vi "XY Graph to Intensity Graph.vi"(8 "error in (no error)":errorcluster, 9 "Y Label":string, 10 "Y Scale":dbl[](array[numeric]), 11 "graph_utilities in":refnum<class "graph_utilities.lvclass">) -> (0 "error out":errorcluster, 3 "graph_utilities out":refnum<class "graph_utilities.lvclass">)   [LabVIEW 2019, in "graph_utilities.lvclass"]
uses:
  graph_utilities.lvclass
  XY Utilities/xy_utilities.lvlib
  XY Utilities/subVIs/Interpolate (multiple).vi
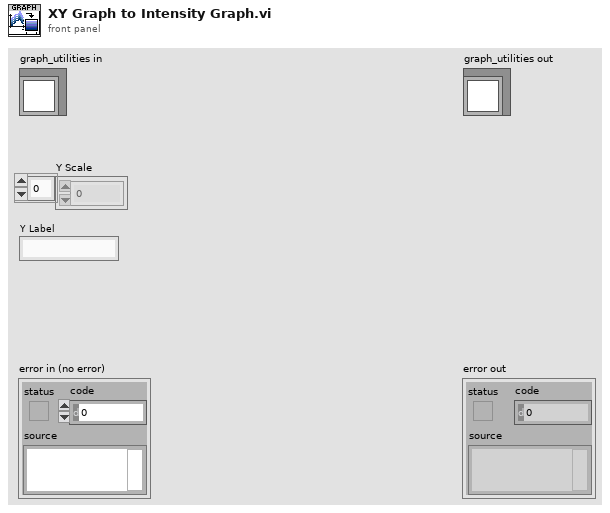
[diagram p1: front panel]
types:
  T1 = cluster{"X Low":dbl, "X High":dbl, "X Step":dbl, "Fake Point":dbl}
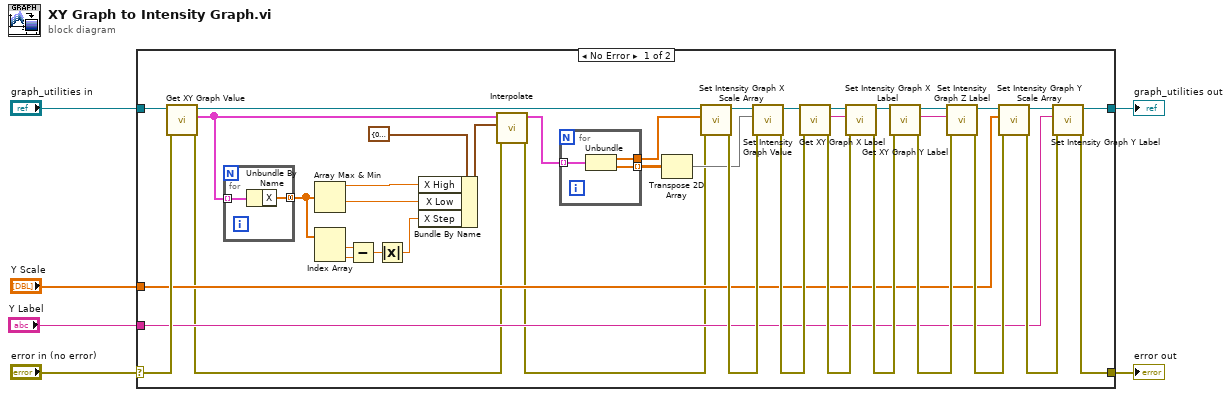
[diagram p0: block diagram]
diagram:
  n1 = case shown="No Error" "error in (no error)" {
    selector: "error in (no error)" -> [w43 w52]
    tunnel: [w25 w52] -> w5
    tunnel: [w33 w51] -> w3
    tunnel: "graph_utilities in" -> [w45 w51]
    tunnel: "Y Scale" -> [w22 _]
    tunnel: "Y Label" -> [w23 _]
    frame No Error {
      n2 = call "Get XY Graph Value.vi"("error in (no error)"=w43, "graph_utilities in"=w45) -> ("error out"=w12:errorcluster, "Value"=w20:cluster{"X":dbl[], "Y":dbl[]}[], "graph_utilities out"=w44:refnum<class "graph_utilities.lvclass">)  [unwired: 7 in]
      n3 = for {
        tunnel: w20 -> [w47] mode=indexing
        tunnel: [w46] -> w10 mode=concatenating
        n4 = Unbundle By Name(w47) -> ("X"=w46:dbl[])
      }
      n5 = Array Max & Min(array=w10) -> (max value=w17:dbl, min value=w18:dbl)  [unwired: 2 out]
      n6 = Index Array(array=w10) -> (element #1=w16:dbl, element #2=w15:dbl)  [unwired: 2 in]
      n7 = Subtract(x=w16, y=w15) -> (x-y=w14:dbl)
      n8 = Absolute Value(x=w14) -> (abs(x)=w9:dbl)
      n9 = Bundle By Name(cluster=T1 {"X Low"=0.05, "X High"=0.5, "X Step"=0.01, "Fake Point"=0.05} ("Configure"), "X High"=w17, "X Low"=w18, "X Step"=w9) -> (w13:T1)
      n10 = call-poly "Interpolate.vi"("error in (no error)"=w12, "Configure"=w13, "XY-data"=w20) -> ("error out"=w11:errorcluster, "Interpolated XY-data out"=w7:cluster{"X-array":dbl[], "Y-array":dbl[]}[])  [unwired: 7 in]
      n11 = for {
        tunnel: w7 -> [w50] mode=indexing
        tunnel: [w49] -> w24 mode=indexing
        tunnel: [w48] -> w8
        n12 = Unbundle(w50) -> ("X-array"=w48:dbl[], "Y-array"=w49:dbl[])
      }
      n13 = Transpose 2D Array(2D array=w24) -> (transposed array=w21:dbl[][])
      n14 = call "Set Intensity Graph X Scale Array.vi"("error in (no error)"=w11, "X Scale"=w8, "graph_utilities in"=w44) -> ("error out"=w32:errorcluster, "graph_utilities out"=w38:refnum<class "graph_utilities.lvclass">)  [unwired: 7 in]
      n15 = call "Set Intensity Graph Value.vi"("error in (no error)"=w32, "Value"=w21, "graph_utilities in"=w38) -> ("error out"=w31:errorcluster, "graph_utilities out"=w37:refnum<class "graph_utilities.lvclass">)  [unwired: 7 in]
      n16 = call "Get XY Graph X Label.vi"("error in (no error)"=w31, "graph_utilities in"=w37) -> ("error out"=w30:errorcluster, "X Label"=w39:string, "graph_utilities out"=w40:refnum<class "graph_utilities.lvclass">)  [unwired: 7 in]
      n17 = call "Set Intensity Graph X Label.vi"("error in (no error)"=w30, "X Label"=w39, "graph_utilities in"=w40) -> ("error out"=w29:errorcluster, "graph_utilities out"=w36:refnum<class "graph_utilities.lvclass">)  [unwired: 7 in]
      n18 = call "Get XY Graph Y Label.vi"("error in (no error)"=w29, "graph_utilities in"=w36) -> ("error out"=w28:errorcluster, "Y Label"=w41:string, "graph_utilities out"=w42:refnum<class "graph_utilities.lvclass">)  [unwired: 7 in]
      n19 = call "Set Intensity Graph Z Label.vi"("error in (no error)"=w28, "Z Label"=w41, "graph_utilities in"=w42) -> ("error out"=w27:errorcluster, "graph_utilities out"=w35:refnum<class "graph_utilities.lvclass">)  [unwired: 7 in]
      n20 = call "Set Intensity Graph Y Scale Array.vi"("error in (no error)"=w27, "Y Scale"=w22, "graph_utilities in"=w35) -> ("error out"=w26:errorcluster, "graph_utilities out"=w34:refnum<class "graph_utilities.lvclass">)  [unwired: 7 in]
      n21 = call "Set Intensity Graph Y Label.vi"("error in (no error)"=w26, "Y Label"=w23, "graph_utilities in"=w34) -> ("error out"=w25:errorcluster, "graph_utilities out"=w33:refnum<class "graph_utilities.lvclass">)  [unwired: 7 in]
    }
    frame Error {
    }
  }
  "error out" <- w5
  "graph_utilities out" <- w3
